vi "Select Device.vi"() -> ()   [LabVIEW 2022 SP3]
uses:
  Global 1.vi
panel:
  in  "cRIO":bool
  in  "cDAQ":bool
  # "Select the Device to Start Accquistion"
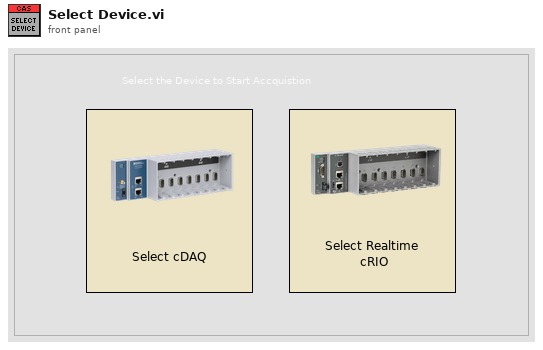
[diagram p1: front panel]
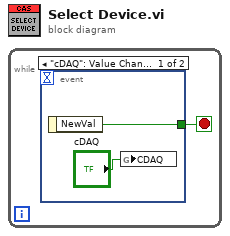
[diagram p0: block diagram]
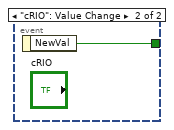
[diagram p2: hidden frame]
diagram:
  n1 = while {
    stop <- w1 stop-if-true
    n2 = event shown="[0] \"cDAQ\": Value Change" {
      selector: _ -> [_ _]
      dyn-events: _ -> [_ _]
      timeout: _ -> [_ _]
      tunnel: [w3 w4] -> w1
      event "cDAQ": Value Change {
        n3 = event-data() -> ("NewVal"=w3:bool)  [unwired: 1 in]
        n4 = global write "Global 1.vi" "CDAQ"("cDAQ") -> ()
      }
      event "cRIO": Value Change {
        n5 = event-data() -> ("NewVal"=w4:bool)  [unwired: 1 in]
      }
    }
  }
